vi "ClassRegistration.vi"() -> ()   [LabVIEW 2020, in "RxnRover.lvlib"]
doc: "Is a non-functional VI which is just used to force register the .lvclasses inside the executable so that LabVIEW always includes them inside the built"
uses:
  RxnRover.lvlib
  Passive Hardware/Passive Hardware.lvclass
  Pump Controller/Pump Controller.lvclass
  Syringe Pump/Syringe Pump.lvclass
  Temperature Controller/Temperature Controller.lvclass
  Parameter to Hardware Map/Parameter to Hardware Map.lvclass
  LC Parser/LC Parser.lvclass
  Generic Optimizer/Generic Optimizer.lvclass
  Controller Array/Controller Array.lvclass
  Controller/Generic Plugin.lvclass
panel:
  in  "RxnRover.lvlib:Generic Plugin.lvclass":refnum<class "Generic Plugin.lvclass">
  in  "RxnRover.lvlib:Controller Array.lvclass":refnum<class "Controller Array.lvclass">
  in  "RxnRover.lvlib:Generic Optimizer.lvclass":refnum<class "Generic Optimizer.lvclass">
  in  "RxnRover.lvlib:LC Parser.lvclass":refnum<class "LC Parser.lvclass">
  in  "RxnRover.lvlib:Parameter to Hardware Map.lvclass":refnum<class "Parameter to Hardware Map.lvclass">
  in  "RxnRover.lvlib:Temperature Controller.lvclass":refnum<class "Temperature Controller.lvclass">
  in  "RxnRover.lvlib:Syringe Pump.lvclass":refnum<class "Syringe Pump.lvclass">
  in  "RxnRover.lvlib:Pump Controller.lvclass":refnum<class "Pump Controller.lvclass">
  in  "RxnRover.lvlib:Passive Hardware.lvclass":refnum<class "Passive Hardware.lvclass">
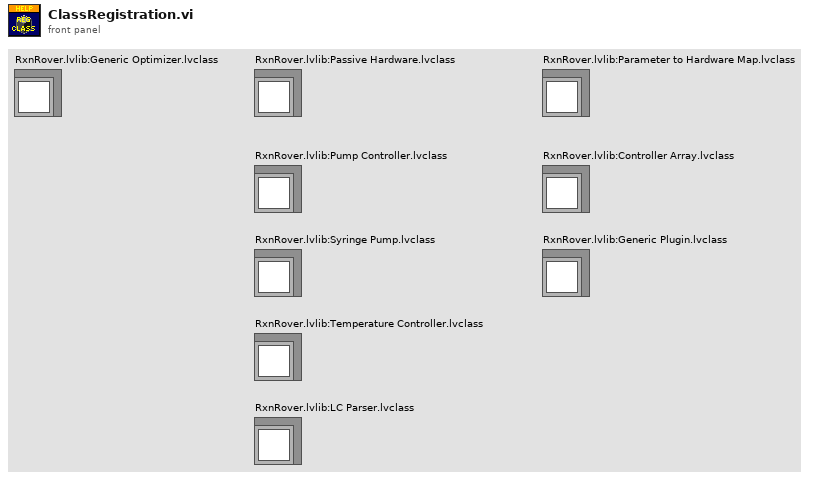
[diagram p1: front panel]
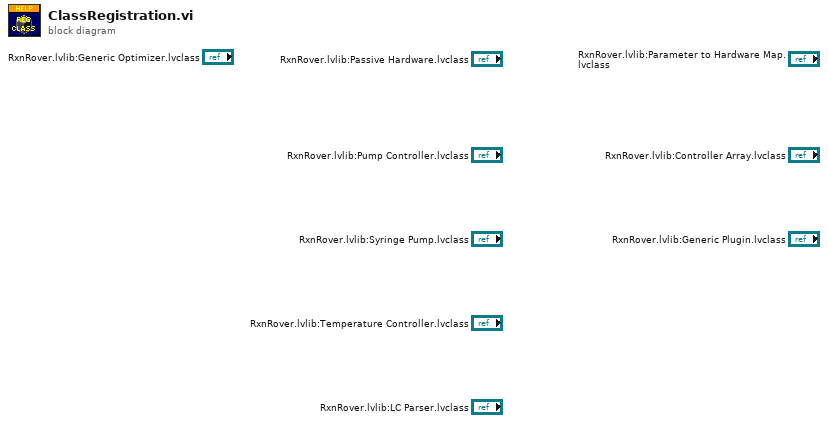
[diagram p0: block diagram]
diagram:
